vi "Gill_get_rdg.vi"(4 "Channel Name":string, 7 "Address":T1={"Main"=67, "Ch."=2, "Sub"=982, "Port Name"="Printer-Modem Port"}) -> (0 "Output":dbl format="%.2f", 1 "Read":string="This is simulation mode", 3 "Status note":string)   [LabVIEW 2014]
uses:
  ADAM Client/Sub VIs/ADAM Controls/Address.ctl
  ADAM Client/Sub VIs/ADAM Controls/Remember_value_mode.ctl
panel:
  out "Concatenated String":string
  out "4521 Address":string
  out "Gill type":i32
  out "ADDRESS LETTER":string
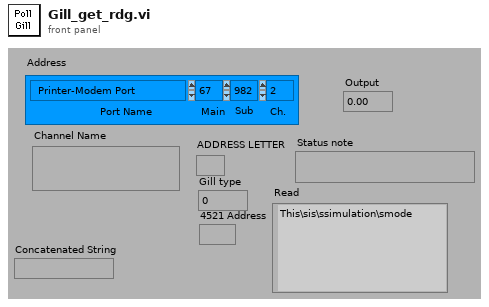
[diagram p1: front panel]
types:
  T1 = typedef "Address.ctl" = cluster{"Main":i32, "Ch.":i32, "Sub":i32, "Port Name":string}
  T2 = typedef "Remember_value_mode.ctl" = enum16{"Read only", "Read and Write"}
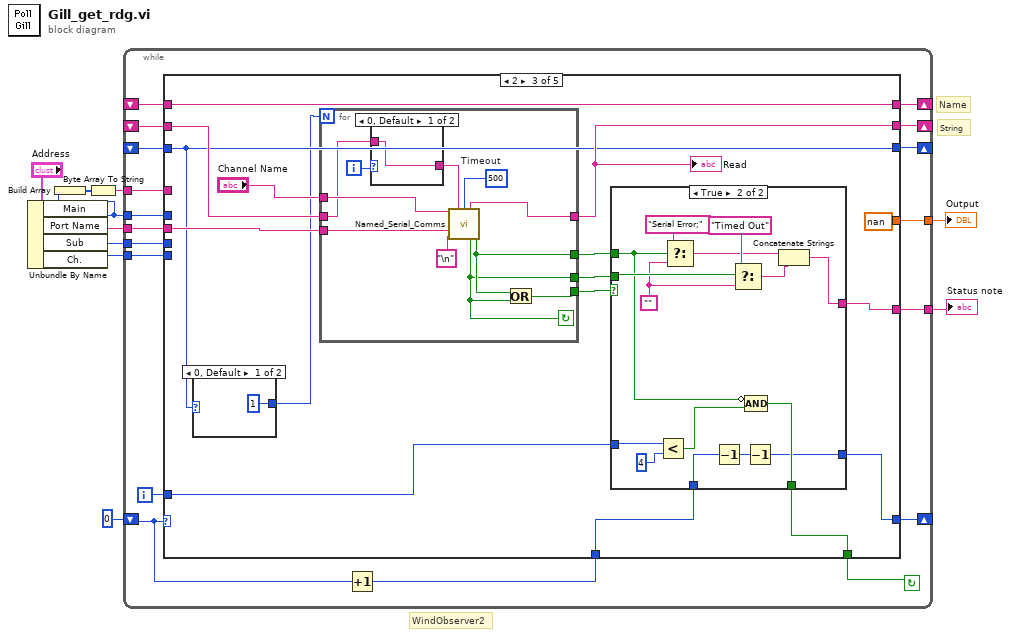
[diagram p0: block diagram]
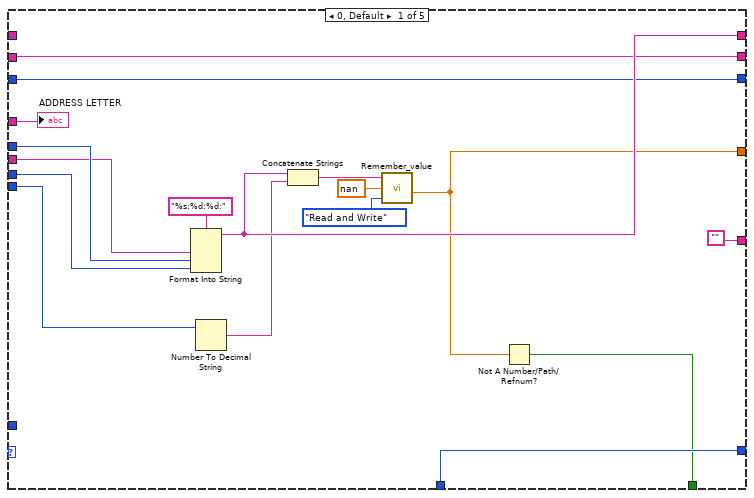
[diagram p2: hidden frame]
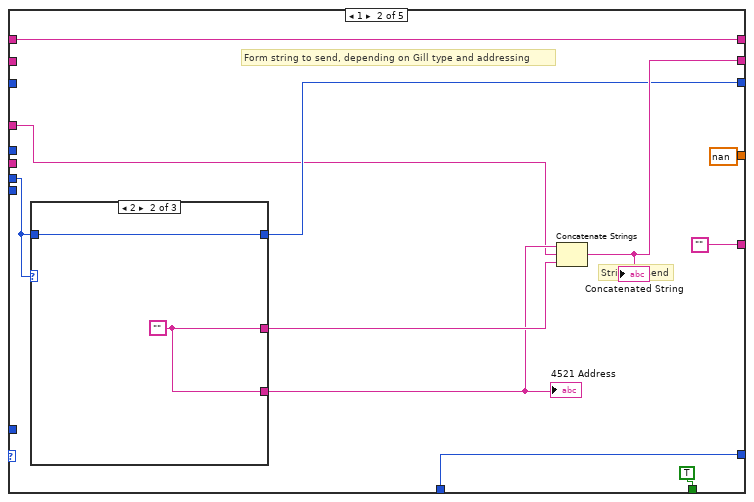
[diagram p3: hidden frame]
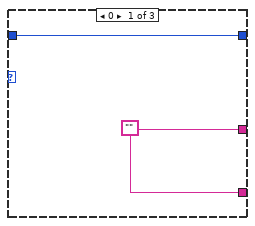
[diagram p4: hidden frame]
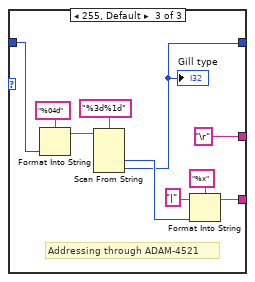
[diagram p5: hidden frame]
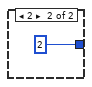
[diagram p6: hidden frame]
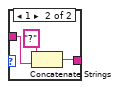
[diagram p7: hidden frame]
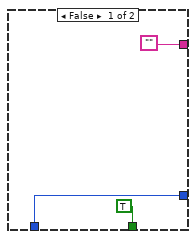
[diagram p8: hidden frame]
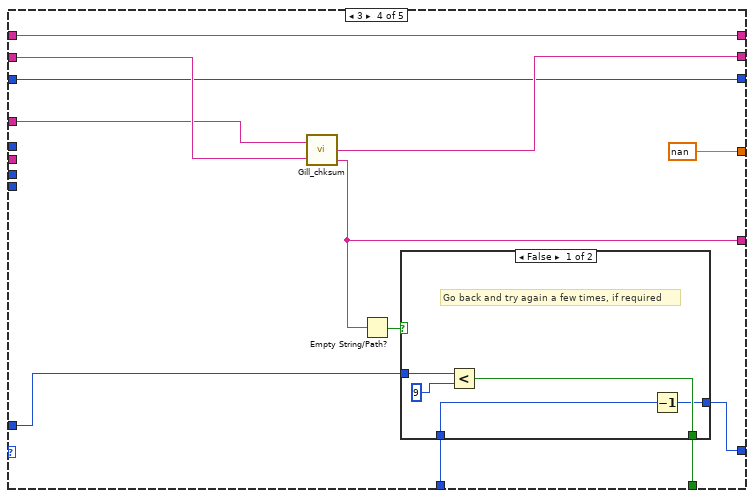
[diagram p9: hidden frame]
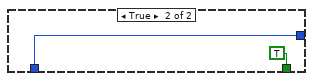
[diagram p10: hidden frame]
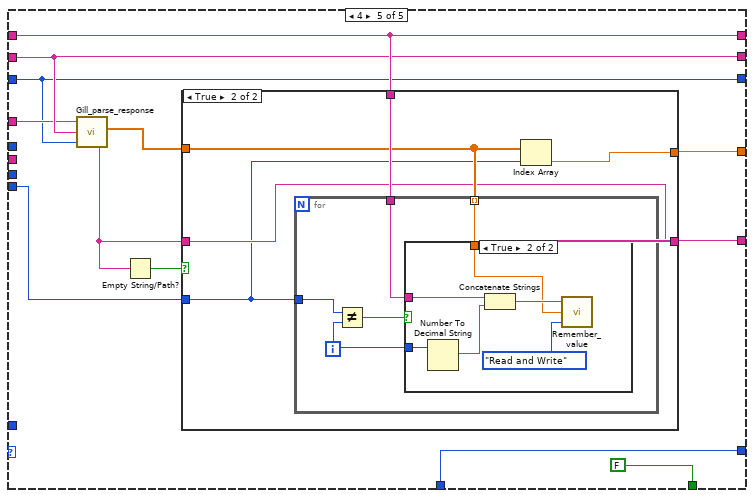
[diagram p11: hidden frame]
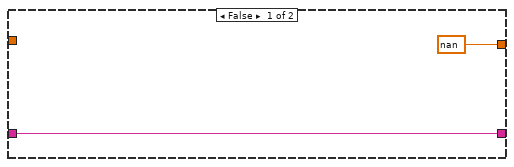
[diagram p12: hidden frame]
diagram:
  # "WindObserver2"
  # "String"
  # "Name"
  n1 = Unbundle By Name("Address") -> ("Main"=w2:i32, "Port Name"=w9:string, "Sub"=w8:i32, "Ch."=w4:i32)
  n2 = Build Array(w2) -> (w3:i32[])
  n3 = Byte Array To String(unsigned byte array=w3) -> (string=w1:string)
  n4 = while {
    shift-left: _ -> [w11]
    shift-right: [w12] -> _
    tunnel: w1 -> [w13]
    shift-left: _ -> [w15]
    shift-right: [w16] -> _
    tunnel: [w19] -> w5
    tunnel: [w20] -> w6
    shift-left: _ -> [w14]
    shift-right: [w21] -> _
    shift-left: 0 -> [w24]
    shift-right: [w22] -> _
    tunnel: w4 -> [w25]
    tunnel: w2 -> [w26]
    tunnel: w8 -> [w27]
    tunnel: w9 -> [w28]
    i -> [w17]
    stop <- w18 continue-if-true
    n5 = Increment(x=w24) -> (x+1=w23:i32)
    n6 = case shown="2" w24 {
      tunnel: w28 -> [w31 _ w85 _ _]
      tunnel: w27 -> [w44 w53 _ _ _]
      tunnel: w26 -> [w45 _ _ _ _]
      tunnel: w25 -> [w42 _ _ _ w145]
      tunnel: w23 -> [w36 w47 w81 w124 w151]
      tunnel: [w36 w47 w80 w125 w151] -> w22
      tunnel: [w41 w54 w76 w130 w144] -> w21
      tunnel: [w33 nan nan nan w146] -> w20
      tunnel: ["" "" w84 w129 w152] -> w19
      tunnel: [w32 TRUE w78 w123 FALSE] -> w18
      tunnel: w17 -> [_ _ w79 w127 _]
      tunnel: [w35 w52 w77 w131 w143] -> w16
      tunnel: w15 -> [w35 _ w73 w132 w143]
      tunnel: w14 -> [_ w54 w76 w130 w144]
      tunnel: w13 -> [w30 w46 _ w128 w142]
      tunnel: [w29 w51 w72 w122 w141] -> w12
      tunnel: w11 -> [w29 _ w72 w122 w141]
      frame 0, Default {
        n7 = Format Into String(format string="%s:%d:%d:" ("Format String"), w31, w45, w44) -> (resulting string=w41:string)  [unwired: 2 in, 1 out]
        n8 = Number To Decimal String(number=w42) -> (decimal integer string=w40:string)  [unwired: 1 out]
        n9 = Concatenate Strings(w41, w40) -> (w39:string)
        n10 = call "Remember_value.vi"("Mode"=Remember_value_mode."Read and Write", "Input Value"=nan, "Ch name"=w39) -> ("Output Value"=w33:dbl)
        n11 = Not A Number/Path/Refnum?(number/path/refnum=w33) -> (NaN/Path/Refnum?=w32:bool)
        "ADDRESS LETTER" <- w30
      }
      frame 1 {
        # "Form string to send, depending on Gill type and addressing"
        # "String to send"
        n12 = case shown="2" w53 {
          tunnel: [w58 w60 w61] -> w51
          tunnel: w53 -> [w58 w60 w70]
          tunnel: [w57 w59 w65] -> w49
          tunnel: [w57 w59 "\r"] -> w50
          frame 0 {
            w57 = ""
          }
          frame 2 {
            w59 = ""
          }
          frame 255, Default {
            # "Addressing through ADAM-4521"
            n13 = Format Into String(format string="%04d" ("Format String"), w70) -> (resulting string=w64:string)  [unwired: 2 in, 1 out]
            n14 = Scan From String(format string="%3d%1d" ("Format String"), input string=w64) -> (output 1=w62:i32, output 2=w61:i32)  [unwired: 2 in, 5 out]
            "Gill type" <- w61
            n15 = Format Into String(format string="%x" ("Format String"), initial string="|" ("Substring"), w62) -> (resulting string=w65:string)  [unwired: 1 in, 1 out]
          }
        }
        "4521 Address" <- w49
        n16 = Concatenate Strings(w49, w46, w50) -> (w52:string)
        "Concatenated String" <- w52
      }
      frame 2 {
        n17 = case shown="0, Default" w72 {
          tunnel: [1 2] -> w71
          frame 0, Default {
          }
          frame 2 {
          }
        }
        n18 = for {
          N: w71 -> [_]
          tunnel: w85 -> [w97]
          tunnel: [w96] -> w82
          tunnel: [w94] -> w75
          tunnel: [w92] -> w74
          tunnel: w73 -> [w90]
          tunnel: "Channel Name" -> [w98]
          tunnel: [w95] -> w77
          i -> [w91]
          stop <- w92 continue-if-true
          w99 = u32 500  # Timeout
          n19 = case shown="0, Default" w91 {
            tunnel: w90 -> [w100 w102]
            tunnel: [w100 w101] -> w89
            frame 0, Default {
            }
            frame 1 {
              n20 = Concatenate Strings("?" ("Substring"), w102) -> (w101:string)
            }
          }
          n21 = call "Named_Serial_Comms.vi"("Channel Name"=w98, "Write String"=w89, "Timeout/ms"=w99, "Port Name"=w97, "Term Grep"="\n") -> ("Read"=w95:string, "Timed out"=w92:bool, "Serial Error"=w94:bool)  [unwired: 4 in, 4 out]
          n22 = Or(x=w94, y=w92) -> (x .or. y?=w96:bool)
        }
        "Read" <- w77
        n23 = case shown="True" w82 {
          tunnel: ["" w120] -> w84
          tunnel: w75 -> [_ w109]
          tunnel: w74 -> [_ w121]
          tunnel: w81 -> [w105 w114]
          tunnel: [w105 w107] -> w80
          tunnel: w79 -> [_ w112]
          tunnel: [TRUE w108] -> w78
          frame False {
          }
          frame True {
            w115 = ""
            n24 = Less?(x=w112, y=4) -> (x < y?=w110:bool)
            n25 = Select(t="Serial Error;", s=w109, f=w115) -> (s? t:f=w117:string)
            n26 = Decrement(x=w114) -> (x-1=w113:i32)
            n27 = Select(t="Timed Out", s=w121, f=w115) -> (s? t:f=w116:string)
            n28 = Compound Arithmetic op=AND(invert w109, w110) -> (w108:bool)
            n29 = Decrement(x=w113) -> (x-1=w107:i32)
            n30 = Concatenate Strings(w117, w116) -> (w120:string)
          }
        }
      }
      frame 3 {
        n31 = call "Gill_chksum.vi"("Address"=w128, "Gill string"=w132) -> ("Stripped string"=w131:string, "Error Notes"=w129:string)  [unwired: 1 out]
        n32 = Empty String/Path?(string/path=w129) -> (empty?=w126:bool)
        n33 = case shown="False" w126 {
          tunnel: w127 -> [w137 _]
          tunnel: [w136 TRUE] -> w123
          tunnel: [w134 w139] -> w125
          tunnel: w124 -> [w135 w139]
          frame False {
            # "Go back and try again a few times, if required"
            n34 = Less?(x=w137, y=9) -> (x < y?=w136:bool)
            n35 = Decrement(x=w135) -> (x-1=w134:i32)
          }
          frame True {
          }
        }
      }
      frame 4 {
        n36 = call "Gill_parse_response.vi"("Address letter"=w142, "Stripped Gill response"=w143, "GILL TYPE NO."=w141) -> ("Numerics"=w150:dbl[], "Error notes"=w149:string)  [unwired: 2 out]
        n37 = Empty String/Path?(string/path=w149) -> (empty?=w148:bool)
        n38 = case shown="True" w148 {
          tunnel: [w153 w156] -> w152
          tunnel: w150 -> [_ w157]
          tunnel: [nan w159] -> w146
          tunnel: w149 -> [w153 w156]
          tunnel: w145 -> [_ w155]
          tunnel: w144 -> [_ w158]
          frame False {
          }
          frame True {
            n39 = for {
              tunnel: w158 -> [w164]
              tunnel: w157 -> [w163] mode=indexing
              tunnel: w155 -> [w161]
              i -> [w162]
              n40 = Not Equal?(x=w161, y=w162) -> (x != y?=w160:bool)
              n41 = case shown="True" w160 {
                tunnel: w162 -> [_ w170]
                tunnel: w164 -> [_ w168]
                tunnel: w163 -> [_ w165]
                frame False {
                }
                frame True {
                  n42 = Number To Decimal String(number=w170) -> (decimal integer string=w169:string)  [unwired: 1 out]
                  n43 = Concatenate Strings(w168, w169) -> (w166:string)
                  n44 = call "Remember_value.vi"("Mode"=Remember_value_mode."Read and Write", "Input Value"=w165, "Ch name"=w166) -> ()  [unwired: 1 out]
                }
              }
            }
            n45 = Index Array(array=w157, index=w155) -> (element=w159:dbl)
          }
        }
      }
    }
  }
  "Output" <- w6
  "Status note" <- w5
